vi "Can Sat.vi"() -> ()   [LabVIEW 2015]
uses:
  <vilib>/Instr/_visa.llb/VISA Configure Serial Port (Instr).vi
panel:
  out "Array":string[](array[string])
  out "XY Graph":cluster{dbl[], dbl[]}(graph)
  out "Longitude":string
  out "Height":string
  out "UV Level":dbl(knob) scale=0.0..10.0
  out "Dust Level":dbl(knob) scale=0.0..600.0
  out "Air Quality(CO)":dbl(knob) scale=0.0..1000.0
  out "Humidity":dbl(slide) scale=0.0..100.0
  out "Temperature":dbl(slide) scale=0.0..100.0
  out "Latitude":string
  out "Time":string
  in  "stop":bool
  out "Raw Data":string
  in  "VISA resource name":refnum<visa-resource-name>
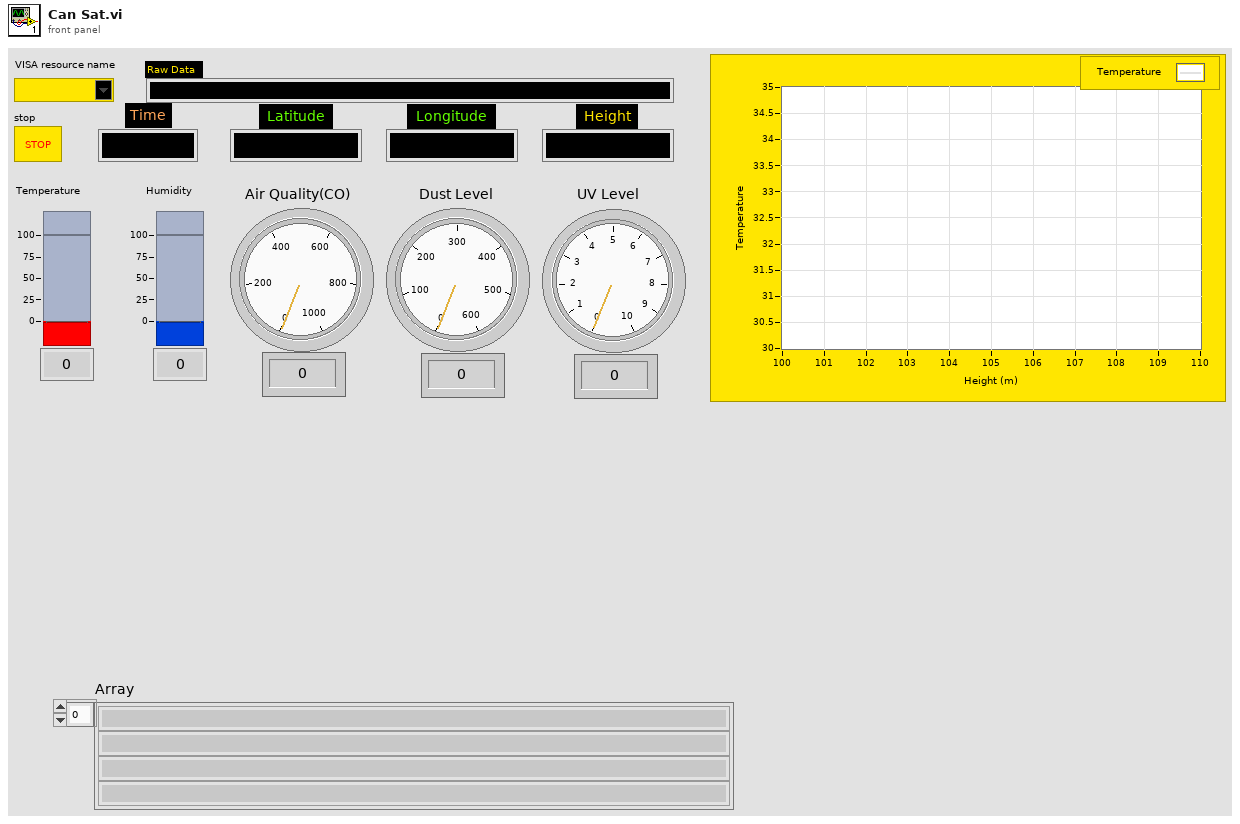
[diagram p1: front panel]
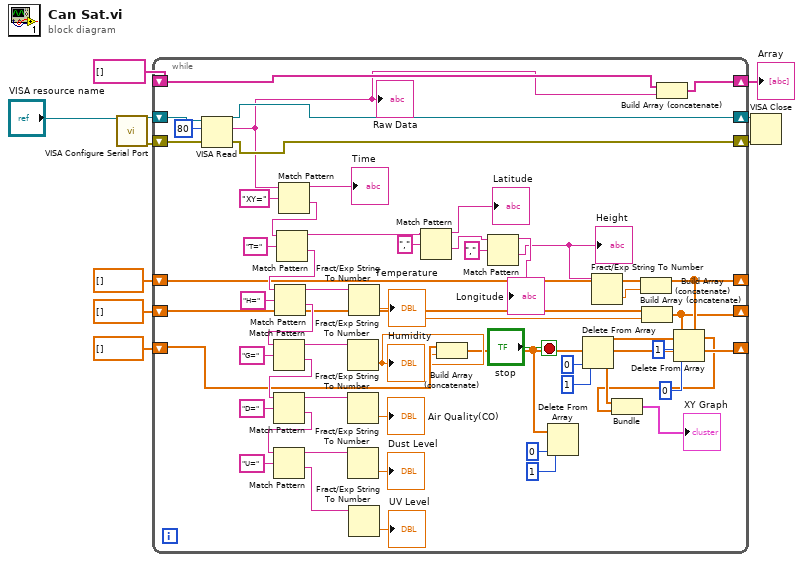
[diagram p0: block diagram]
diagram:
  n1 = call-poly "VISA Configure Serial Port"("VISA resource name"="VISA resource name") -> ("VISA resource name out"=w9:refnum<visa-resource-name>, "error out"=w8:errorcluster)  [unwired: 13 in]
  n2 = while {
    shift-right: [w61] -> w7
    shift-left: w9 -> [w64]
    shift-right: [w60] -> w6
    shift-left: w8 -> [w63]
    shift-right: [w27] -> _
    shift-left: dbl[] [] -> [w31]
    shift-right: [w26] -> _
    shift-left: dbl[] [] -> [w29]
    shift-right: [w20] -> w1
    shift-left: string[] [] -> [w19]
    shift-right: [w13] -> _
    shift-left: dbl[] [] -> [w17]
    stop <- "stop" stop-if-true
    n3 = VISA Read(VISA resource name=w64, byte count=u32 80, error in (no error)=w63) -> (VISA resource name out=w61:refnum<visa-resource-name>, read buffer=w18:string, error out=w60:errorcluster)  [unwired: 1 out]
    "Raw Data" <- w18
    n4 = Match Pattern(string=w18, regular expression="XY=") -> (before substring=→"Time":string, after substring=w55:string)  [unwired: 1 in, 2 out]
    n5 = Match Pattern(string=w55, regular expression="T=") -> (before substring=w38:string, after substring=w53:string)  [unwired: 1 in, 2 out]
    n6 = Match Pattern(string=w53, regular expression="H=") -> (before substring=w52:string, after substring=w49:string)  [unwired: 1 in, 2 out]
    n7 = Match Pattern(string=w49, regular expression="G=") -> (before substring=w50:string, after substring=w45:string)  [unwired: 1 in, 2 out]
    n8 = Match Pattern(string=w45, regular expression="D=") -> (before substring=w47:string, after substring=w40:string)  [unwired: 1 in, 2 out]
    n9 = Match Pattern(string=w40, regular expression="U=") -> (before substring=w43:string, after substring=w39:string)  [unwired: 1 in, 2 out]
    n10 = Fract/Exp String To Number(string=w50) -> (number=w16:dbl)  [unwired: 3 in, 1 out]
    "Humidity" <- w16
    n11 = Fract/Exp String To Number(string=w47) -> (number=→"Air Quality(CO)":dbl)  [unwired: 3 in, 1 out]
    n12 = Fract/Exp String To Number(string=w43) -> (number=→"Dust Level":dbl)  [unwired: 3 in, 1 out]
    n13 = Fract/Exp String To Number(string=w52) -> (number=w28:dbl)  [unwired: 3 in, 1 out]
    "Temperature" <- w28
    n14 = Fract/Exp String To Number(string=w39) -> (number=→"UV Level":dbl)  [unwired: 3 in, 1 out]
    n15 = Match Pattern(string=w38, regular expression=",") -> (before substring=→"Latitude":string, after substring=w35:string)  [unwired: 1 in, 2 out]
    n16 = Build Array (concatenate)(w17, w16) -> (w13:dbl[])
    n17 = Match Pattern(string=w35, regular expression=",") -> (before substring=→"Longitude":string, after substring=w32:string)  [unwired: 1 in, 2 out]
    "Height" <- w32
    n18 = Delete From Array(array=w13, length=1, index=0) -> ()  [unwired: 2 out]
    n19 = Fract/Exp String To Number(string=w32) -> (number=w30:dbl)  [unwired: 3 in, 1 out]
    n20 = Build Array (concatenate)(w31, w30) -> (w27:dbl[])
    n21 = Delete From Array(array=w27, length=1, index=0) -> (array with subset deleted=w25:dbl[])  [unwired: 1 out]
    n22 = Build Array (concatenate)(w29, w28) -> (w26:dbl[])
    n23 = Build Array (concatenate)(w19, w18) -> (w20:string[])
    n24 = Delete From Array(array=w26, length=1, index=0) -> (array with subset deleted=w11:dbl[])  [unwired: 1 out]
    n25 = Bundle(w25, w11) -> (→"XY Graph":cluster{dbl[], dbl[]})  [unwired: 1 in]
  }
  "Array" <- w1
  n26 = VISA Close(VISA resource name=w7, error in (no error)=w6) -> ()  [unwired: 1 out]
